vi "Read Message.vi"(8 "error in (no error)":errorcluster, 9 "timeout":i32, 11 "TCPIP in":refnum<class "TCPIP.lvclass">) -> (0 "error out":errorcluster, 2 "Message":string, 3 "TCPIP out":refnum<class "TCPIP.lvclass">)   [LabVIEW 2018, in "TCPIP.lvclass"]
uses:
  TCPIP.lvclass
  TCPIP.lvclass/TCPIP.ctl
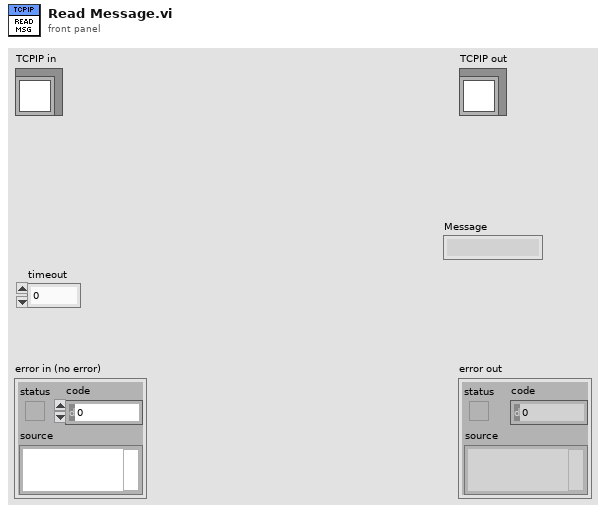
[diagram p1: front panel]
types:
  T1 = enum16{"Standard", "Buffered", "CRLF", "Immediate"}
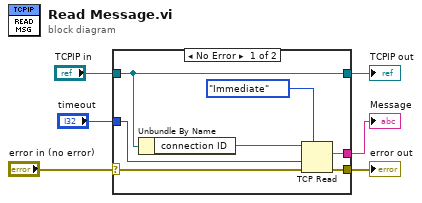
[diagram p0: block diagram]
diagram:
  n1 = case shown="No Error" "error in (no error)" {
    selector: "error in (no error)" -> [w13 w15]
    tunnel: [w12 w15] -> w5
    tunnel: [w11 w14] -> w3
    tunnel: "TCPIP in" -> [w11 w14]
    tunnel: [w9 _] -> w2
    tunnel: "timeout" -> [w8 _]
    frame No Error {
      n2 = Unbundle By Name(w11) -> ("connection ID"=w10:refnum<k5>)
      n3 = TCP Read(connection ID=w10, error in (no error)=w13, 7:T1."Immediate" ("mode (standard)"), 9:w8) -> (data out=w9:string, error out=w12:errorcluster)  [unwired: 1 in, 1 out]
    }
    frame Error {
    }
  }
  "error out" <- w5
  "TCPIP out" <- w3
  "Message" <- w2
